vi "peak detect, max.vi"(5 "timetrace":dbl[](array[numeric]), 9 "threshold":dbl) -> (6 "locations":dbl[](array[numeric]), 10 "amplitudes":dbl[](array[numeric]))   [LabVIEW 2009]
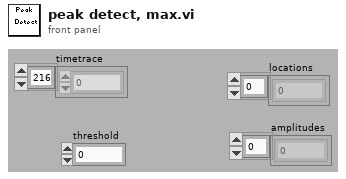
[diagram p1: front panel]
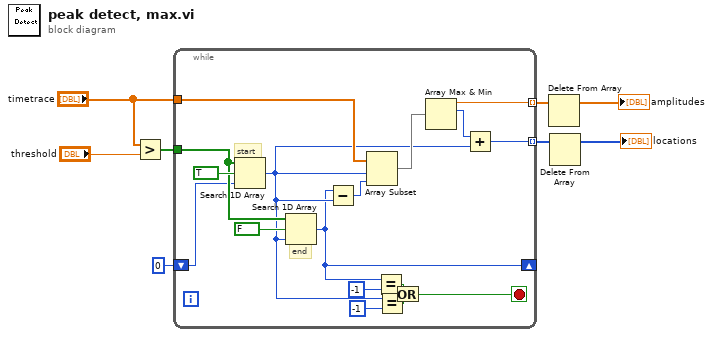
[diagram p0: block diagram]
diagram:
  n1 = Greater?(x="timetrace", y="threshold") -> (0:w4:bool[])
  n2 = while {
    tunnel: w4 -> [w23]
    tunnel: "timetrace" -> [w21]
    tunnel: [w18] -> w2 mode=indexing
    tunnel: [w17] -> w3 mode=indexing
    shift-right: [w12] -> _
    shift-left: 0 ("index of element") -> [w16]
    stop <- w9 stop-if-true
    # "end"
    # "start"
    n3 = Search 1D Array(1D array=w23, element=TRUE, start index (0)=w16) -> (index of element=w15:i32)
    n4 = Search 1D Array(1D array=w23, element=FALSE, start index (0)=w15) -> (index of element=w12:i32)
    n5 = Subtract(x=w12, y=w15) -> (x-y=w22:i32)
    n6 = Array Subset(array=w21, index=w15, length=w22) -> (w20:dbl[])
    n7 = Equal?(x=w12, y=-1) -> (x = y?=w10:bool)
    n8 = Equal?(x=w15, y=-1) -> (x = y?=w11:bool)
    n9 = Or(x=w10, y=w11) -> (x .or. y?=w9:bool)
    n10 = Array Max & Min(array=w20) -> (max value=w18:dbl, max index (indices)=w19:i32)  [unwired: 2 out]
    n11 = Add(x=w19, y=w15) -> (x+y=w17:i32)
  }
  n12 = Delete From Array(array=w2) -> (array with subset deleted=→"amplitudes":dbl[])  [unwired: 2 in, 1 out]
  n13 = Delete From Array(array=w3) -> (array with subset deleted=→"locations":i32[])  [unwired: 2 in, 1 out]
